vi "RPC.vi"(0 "mbed_LVLibrary.lvlib:SerialRPC.lvclass":refnum<class "SerialRPC.lvclass">, 5 "Name":string, 7 "method":string, 9 "Args":string[](array[string]), 11 "error in (no error)":errorcluster) -> (4 "mbed_LVLibrary.lvlib:SerialRPC.lvclass 2":refnum<class "SerialRPC.lvclass">, 8 "RPC Result":string, 15 "error out":errorcluster)   [LabVIEW 2011, in "mbed_LVLibrary.lvlib" / "SerialRPC.lvclass"]
doc: "This VI implements the RPC over serial, this VI should not be used in applications. It is a dynamic instance and so the RPC function within the mbed class should be used. This will make it possible to change the method of communicating with mbed without needing to make many changes to your application"
uses:
  SerialRPC.lvclass
  <vilib>/Instr/_visa.llb/VISA Flush IO Buffer Mask.ctl
  SerialRPC.lvclass/SerialRPC.ctl
  mbed/mbed.lvclass
panel:
  out "The RPC string":string
  out "Read Return count":u32
  out "return count":u32
  # "Write the RPC data over serial"
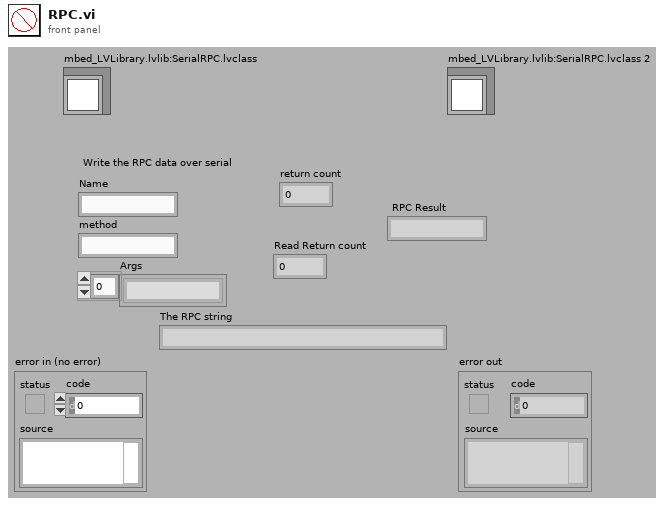
[diagram p1: front panel]
types:
  T1 = typedef "VISA Flush IO Buffer Mask.ctl" = u16
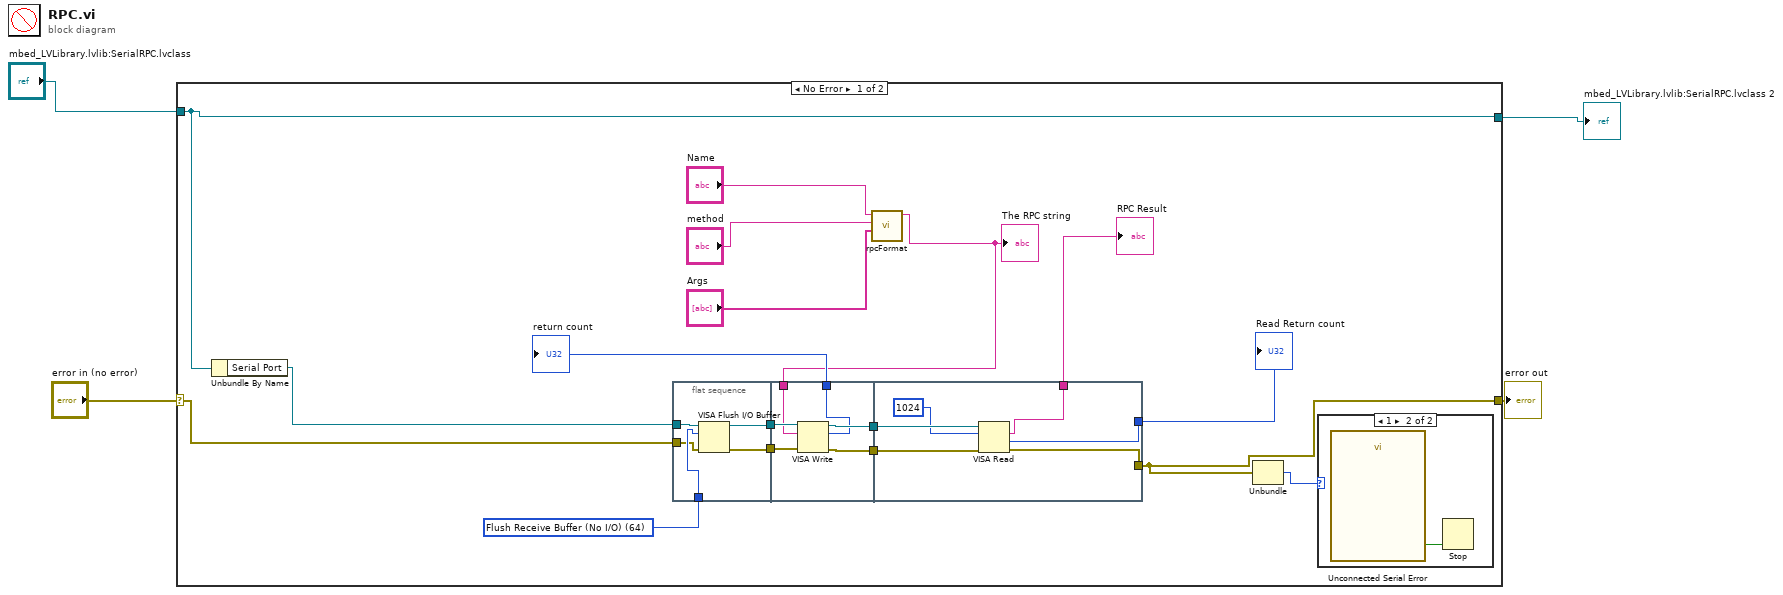
[diagram p0: block diagram]
diagram:
  n1 = case shown="No Error" "error in (no error)" {
    selector: "error in (no error)" -> [w12 w41]
    tunnel: [w14 w41] -> w3
    tunnel: [w10 w40] -> w2
    tunnel: "mbed_LVLibrary.lvlib:SerialRPC.lvclass" -> [w10 w40]
    frame No Error {
      w15 = T1 64 items=["Flush Receive Buffer"=16, "Write Transmit Buffer to Device"=32, "Flush Receive Buffer (No I/O)"=64, "Flush Transmit Buffer"=128] ("Mask")
      n2 = Unbundle By Name(w10) -> ("Serial Port"=w5:refnum<visa-resource-name>)
      n3 = flat-sequence {
        tunnel: w5 -> [w27]
        tunnel: w15 -> [w24]
        tunnel: [w25] -> w21
        tunnel: [w26] -> w20
        tunnel: w12 -> [w23]
        tunnel: [w33] -> w19
        tunnel: [w32] -> w18
        tunnel: [w31] -> w17
        tunnel: w21 -> [w30]
        tunnel: w20 -> [w29]
        tunnel: w6 -> [w28]
        tunnel: w19 -> [w39]
        tunnel: [w38] -> w11
        tunnel: w18 -> [w37]
        tunnel: [w36] -> w14
        tunnel: [w35] -> w16
        frame #0 {
          n4 = VISA Flush I/O Buffer(VISA resource name=w27, mask (16)=w24, error in (no error)=w23) -> (VISA resource name out=w26:refnum<visa-resource-name>, error out=w25:errorcluster)
        }
        frame #1 {
          n5 = VISA Write(VISA resource name=w29, write buffer=w28, error in (no error)=w30) -> (VISA resource name out=w33:refnum<visa-resource-name>, return count=w31:u32, error out=w32:errorcluster)
        }
        frame #2 {
          n6 = VISA Read(VISA resource name=w39, byte count=u32 1024, error in (no error)=w37) -> (read buffer=w38:string, return count=w35:u32, error out=w36:errorcluster)  [unwired: 1 out]
        }
      }
      n7 = call "rpcFormat.vi"("Args"="Args", "method"="method", "Name"="Name") -> ("The RPC string"=w6:string)  [unwired: 8 in]
      "The RPC string" <- w6
      n8 = Unbundle(w14) -> ("code"=w13:i32)  [unwired: 2 out]
      n9 = case shown="1" w13 {
        frame 0, Default {
        }
        frame 1 {
          n10 = call "Unconnected Serial Error"() -> ("OK"=w22:bool)  [unwired: 10 in, 1 out]
          n11 = Stop(stop? (T)=w22) -> ()
        }
      }
      "return count" <- w17
      "Read Return count" <- w16
      "RPC Result" <- w11
    }
    frame Error {
    }
  }
  "error out" <- w3
  "mbed_LVLibrary.lvlib:SerialRPC.lvclass 2" <- w2
